vi "Decode_SignedHundredths.vi"(1 "Little Endian":u8[](array[numeric])) -> (0 "Signed Hundredths (0.00)":dbl[](array[numeric]))   [LabVIEW 2015, in "navX Library v3.lvlib" / "navX Registry Cache.lvclass"]
uses:
  navX Registry Cache.lvclass
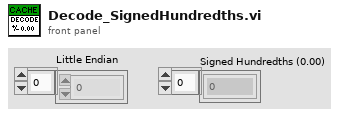
[diagram p1: front panel]
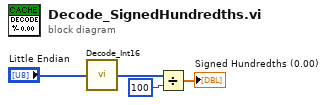
[diagram p0: block diagram]
diagram:
  n1 = call "Decode_Int16.vi"("Little Endian"="Little Endian") -> ("Int16"=w2:i16[])
  n2 = Divide(x=w2, y=100) -> (x/y=→"Signed Hundredths (0.00)":dbl[])
